vi "SetTriggerDelay.vi"(8 "error in (no error)":errorcluster, 10 "Arg":string, 11 "Point Grey Camera in":refnum<class "Point Grey Camera.lvclass">) -> (0 "error out":errorcluster, 2 "setValue out":dbl, 3 "Point Grey Camera out":refnum<class "Point Grey Camera.lvclass">)   [LabVIEW 2020, in "Point Grey Camera.lvclass"]
uses:
  Point Grey Camera.lvclass
  Point Grey Camera.lvclass/Point Grey Camera.ctl
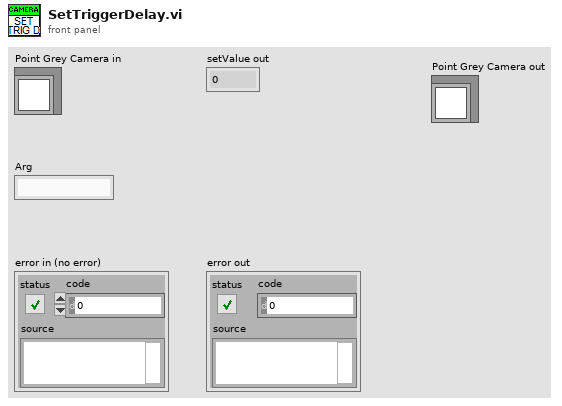
[diagram p1: front panel]
types:
  T1 = typedef "IMAQdx.ctl" = refnum<k21>
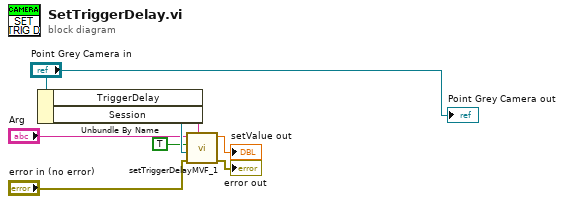
[diagram p0: block diagram]
diagram:
  n1 = Unbundle By Name("Point Grey Camera in") -> ("TriggerDelay"=w8:string, "Session"=w5:T1)
  n2 = call "setTriggerDelayMVF_1.vi"("TriggerDelayName"=w8, "error in"="error in (no error)", "Session"=w5, "CAM connected"=TRUE, "setValue"="Arg") -> ("error out"=→"error out":errorcluster, "setValue out"=→"setValue out":dbl)  [unwired: 2 in]
  "Point Grey Camera out" <- "Point Grey Camera in"
